vi "SLAMTest.vi"() -> ()   [LabVIEW 2009, in "Test.lvlib"]
uses:
  Test.lvlib
  Main.lvlib
panel:
  out "error out":errorcluster
  out "Xout":dbl[](array[numeric])
  in  "deltaPosition":cluster{"X":dbl, "Y":dbl, "Angle":dbl}
  in  "Walls":T1(array[cluster])
  in  "stop":bool
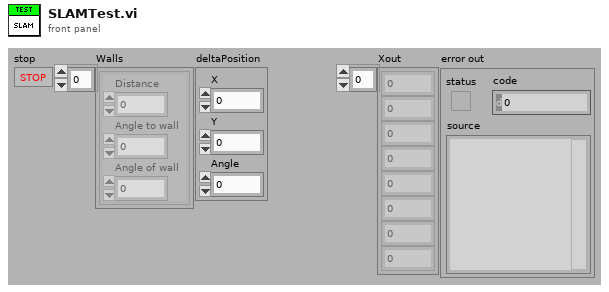
[diagram p1: front panel]
types:
  T1 = cluster{"Distance":dbl, "Angle to wall":dbl, "Angle of wall":dbl}[]
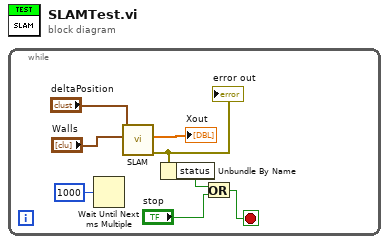
[diagram p0: block diagram]
diagram:
  n1 = while {
    stop <- w3 stop-if-true
    n2 = Wait Until Next ms Multiple(millisecond multiple=u32 1000) -> ()  [unwired: 1 out]
    n3 = call "SLAM.vi"("deltaPosition"="deltaPosition", "Walls"="Walls") -> ("error out"=w2:errorcluster, "Xout"=→"Xout":dbl[])  [unwired: 8 in]
    "error out" <- w2
    n4 = Unbundle By Name(w2) -> ("status"=w1:bool)
    n5 = Or(x=w1, y="stop") -> (x .or. y?=w3:bool)
  }
